vi "insertQuery.vi"() -> ()   [LabVIEW 2025]
uses:
  <vilib>/addons/database/Connection.llb/DB Tools Open Connec (String).vi
  <vilib>/addons/database/Connection.llb/Conn Execute.vi
  <vilib>/addons/database/Recordset.llb/Rec Destroy - Connection.vi
  <vilib>/addons/database/NI_Database_API.lvlib
panel:
  in  "Boolean":bool
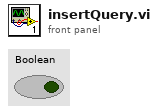
[diagram p1: front panel]
types:
  T1 = typedef "NI_Database_API.lvlib/Conn ObjectReference.ctl" = refnum<k1>
  T2 = typedef "NI_Database_API.lvlib/Rec ObjectReference.ctl" = refnum<k1>
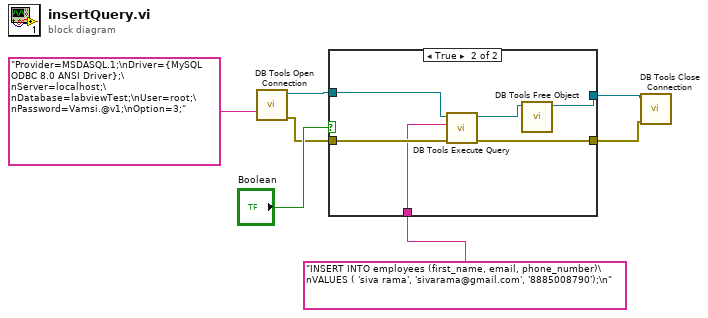
[diagram p0: block diagram]
diagram:
  n1 = call-poly <vilib>:"DB Tools Open Connection.vi"("connection information"="Provider=MSDASQL.1;\nDriver={MySQL ODBC 8.0 ANSI Driver};\nServer=localhost;\nDatabase=labviewTest;\nUser=root;\nPassword=Vamsi.@v1;\nOption=3;") -> ("error out"=w5:errorcluster, "connection reference"=w3:T1)  [unwired: 7 in]
  n2 = case shown="True" "Boolean" {
    tunnel: w5 -> [w8 w15]
    tunnel: "INSERT INTO employees (first_name, email, phone_number)\nVALUES ( 'siva rama', 'sivarama@gmail.com', '8885008790');\n" -> [_ w14]
    tunnel: w3 -> [w9 w13]
    tunnel: [w9 w10] -> w2
    tunnel: [w8 w12] -> w1
    frame False {
    }
    frame True {
      n3 = call-poly <vilib>:"DB Tools Execute Query.vi"("error in (no error)"=w15, "SQL query"=w14, "connection reference"=w13) -> ("error out"=w12:errorcluster, "recordset reference"=w11:T2)  [unwired: 5 in]
      n4 = call-poly <vilib>:"DB Tools Free Object.vi"("recordset reference"=w11) -> ("connection reference"=w10:T1)  [unwired: 9 in, 1 out]
    }
  }
  n5 = call <vilib>:"DB Tools Close Connection.vi"("error in (no error)"=w1, "connection reference"=w2) -> ()  [unwired: 5 in, 1 out]
